vi "Get Power Meter Default Value.vi"(0 "SG Path 568x Accessor in":refnum<class "SG Path Accessor.lvclass">, 11 "error in (no error)":errorcluster) -> (4 "SG Path 568x Accessor out":refnum<class "SG Path Accessor.lvclass">, 6 "Power Meter out":refnum<class "Power Meter Base.lvclass">, 15 "error out":errorcluster)   [LabVIEW 2023, in "NI-568x RF Power Meter.lvlib" / "SG Path Accessor.lvclass"]
uses:
  SG Path Accessor.lvclass
  Instruments/Power Meter/Power Meter Base/Power Meter Base.lvclass
  Power Meter/Power Meter.lvclass
  C:/srd-semi-rfcal-software/AuxTools/STSRFFixtureCharactUtility/Source/Code Modules/Fixture/Instruments/Power Meter/Power Meter Base/Power Meter Base.lvclass
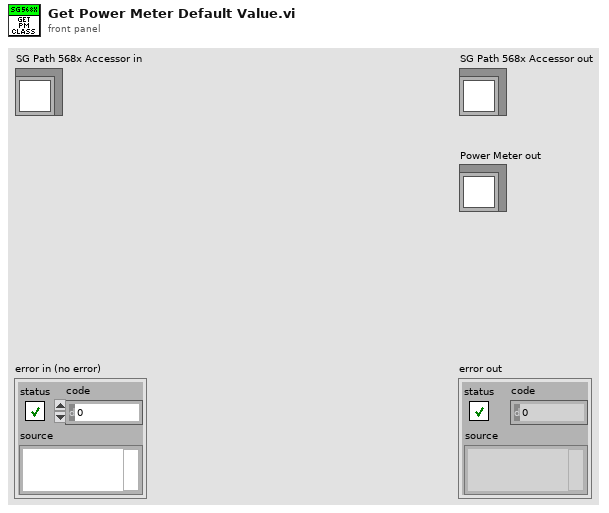
[diagram p1: front panel]
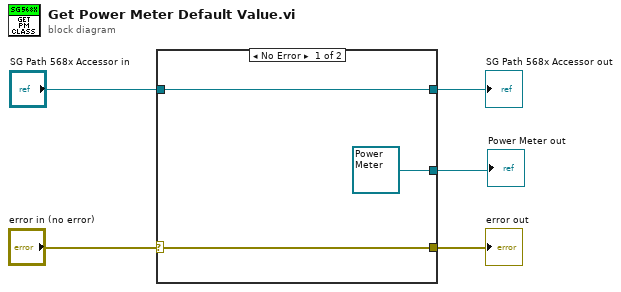
[diagram p0: block diagram]
diagram:
  n1 = case shown="No Error" "error in (no error)" {
    selector: "error in (no error)" -> [w6 w9]
    tunnel: "SG Path 568x Accessor in" -> [w7 w10]
    tunnel: [w7 w10] -> w4
    tunnel: [w6 w9] -> w3
    tunnel: [refnum<class "Power Meter.lvclass"> refnum ("STS Scalar Fixture Charact.lvlib:PM NI568X.lvclass") _] -> w1
    frame No Error {
    }
    frame Error {
    }
  }
  "error out" <- w3
  "SG Path 568x Accessor out" <- w4
  "Power Meter out" <- w1
